vi "SortAnnularScans.vi"(2 "file names":string[](array[string]), 3 "Scan Planes":i32=1, 4 "RootName":string, 6 "Transmit Rings":i8=5, 7 "directory path":path) -> ()   [LabVIEW 2022 SP3]
panel:
  out "file list":string[][][](array[string])
  out "saved files":string[][][](array[string])
  # "Data is always assumed to come in as a set starting with ring 1"
  # "Select number of rings acquired from. Always 5"
  # "Choose number of LeCroy Chans used. Normally 4. If using T/R from ring pairs, set to zero"
  # "Select root file name: i.e. TRTest1a for TRTest1a001.eye"
  # "Results saved as new eye files with format of TRTest1a1to1.eye, TRTest1a1to2.eye, etc. New eye files modify the RF att value in the header to account for the LeCroy attenuation based on the voltage scale. May need to add additional offset if pre-amps are used on LeCroy input. Would also have to adjust for Panametrics gain."
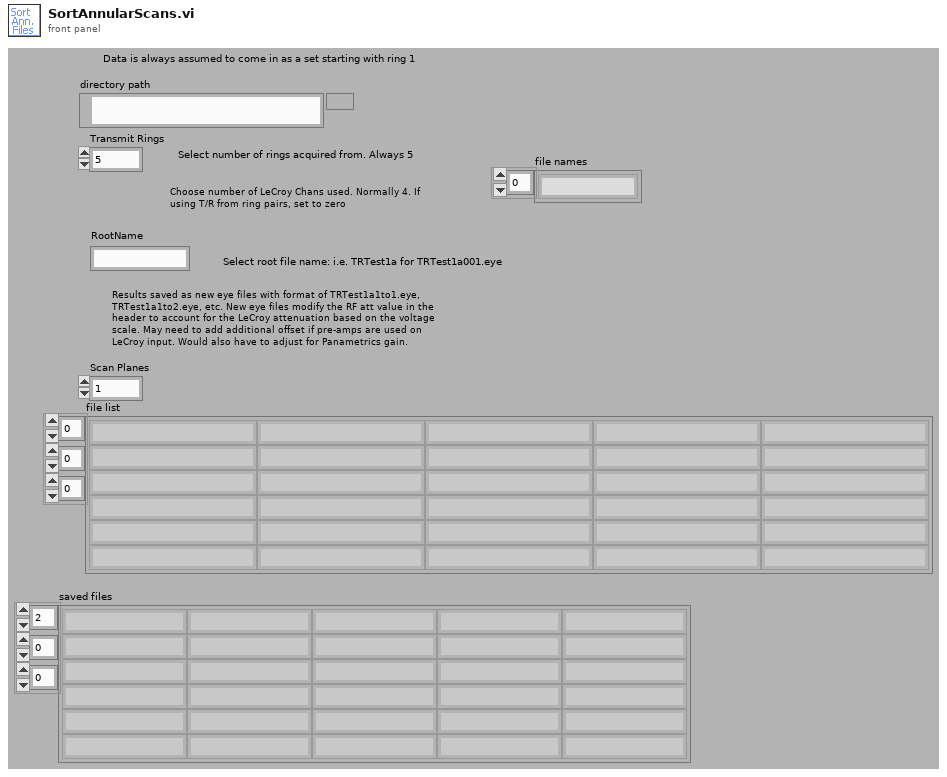
[diagram p1: front panel]
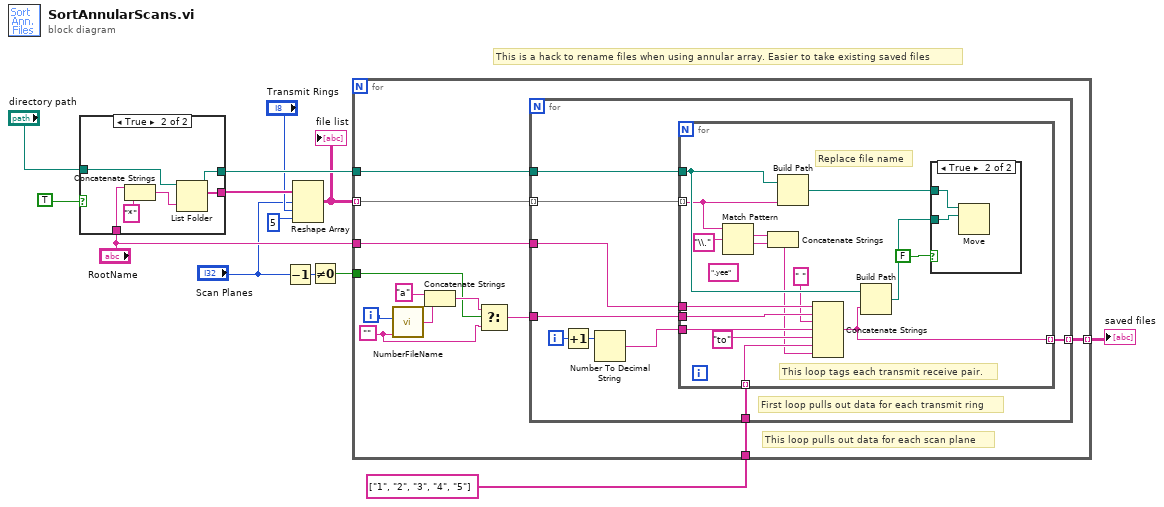
[diagram p0: block diagram]
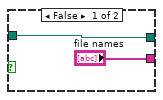
[diagram p3: hidden frame]
diagram:
  # "This is a hack to rename files when using annular array. Easier to take existing saved files"
  n1 = case shown="True" TRUE ("Case Constant\n(See Context Help)") {
    tunnel: [w15 w21] -> w13
    tunnel: ["file names" w20] -> w5
    tunnel: "RootName" -> [_ w19]
    tunnel: "directory path" -> [w15 w16]
    frame False {
    }
    frame True {
      n2 = Concatenate Strings(w19, "*") -> (w17:string)
      n3 = List Folder(path=w16, pattern=w17) -> (path out=w21:path, filenames=w20:string[])  [unwired: 2 in, 2 out]
    }
  }
  n4 = Decrement(x="Scan Planes") -> (x-1=w10:i32)
  n5 = Reshape Array(w5, "Scan Planes", "Transmit Rings", 5) -> (w2:string[][][])
  "file list" <- w2
  n6 = Not Equal To 0?(x=w10) -> (x != 0?=w11:bool)
  n7 = for {
    tunnel: w13 -> [w32]
    tunnel: w2 -> [w33] mode=indexing
    tunnel: "RootName" -> [w31]
    tunnel: w11 -> [w22]
    tunnel: [w30] -> w6 mode=indexing
    tunnel: string[] ["1", "2", "3", "4", "5"] ("transposed array") -> [w29]
    i -> [w23]
    w25 = ""
    # "This loop pulls out data for each scan plane"
    n8 = call "NumberFileName.vi"("String"=w25, "File number"=w23) -> ("Numbered File"=w28:string)  [unwired: 2 in]
    n9 = Concatenate Strings("a", w28) -> (w26:string)
    n10 = Select(t=w26, s=w22, f=w25) -> (s? t:f=w24:string)
    n11 = for {
      tunnel: w33 -> [w42] mode=indexing
      tunnel: w32 -> [w41]
      tunnel: w29 -> [w40]
      tunnel: w31 -> [w39]
      tunnel: [w38] -> w30 mode=indexing
      tunnel: w24 -> [w34]
      i -> [w36]
      # "First loop pulls out data for each transmit ring"
      n12 = Increment(x=w36) -> (x+1=w37:i32)
      n13 = Number To Decimal String(number=w37) -> (decimal integer string=w35:string)  [unwired: 1 in]
      n14 = for {
        tunnel: w42 -> [w48] mode=indexing
        tunnel: w41 -> [w55]
        tunnel: w35 -> [w57]
        tunnel: w40 -> [w56] mode=indexing
        tunnel: w39 -> [w51]
        tunnel: w34 -> [w50]
        tunnel: [w53] -> w38 mode=indexing
        (unwired) ".yee"
        # "Replace file name"
        # "This loop tags each transmit receive pair."
        n15 = Match Pattern(string=w48, regular expression="\\.") -> (match substring=w45:string, after substring=w44:string)  [unwired: 1 in, 2 out]
        n16 = Concatenate Strings(w45, w44) -> (w46:string)
        n17 = Build Path(base path=w55, name or relative path=w48) -> (appended path=w54:path)
        n18 = Concatenate Strings(w51, w50, " ", w57, "to", w56, w46) -> (w53:string)
        n19 = Build Path(base path=w55, name or relative path=w53) -> (appended path=w52:path)
        n20 = case shown="True" FALSE ("Case Constant\n(See Context Help) 2") {
          tunnel: w52 -> [_ w60]
          tunnel: w54 -> [_ w59]
          frame False {
          }
          frame True {
            n21 = Move(source path=w59, 10:w60) -> ()  [unwired: 3 in, 3 out]
          }
        }
      }
    }
  }
  "saved files" <- w6
